vi "CaseStructure - Check If State Exist.vi"(8 "error in (no error)":errorcluster, 10 "Group Name":string, 11 "CaseStructure in":refnum<vi>) -> (0 "error out":errorcluster, 2 "Numeric":i32, 3 "CaseStructure out":refnum<vi>)   [LabVIEW 2017, in "csmHelper-CaseStructure.lvlib"]
doc: "-- <b>输入控件</b> --\n\n- <b>Group Name</b>:\n\n- <b>CaseStructure in</b>:\n\n-- <b>输出控件</b> --\n\n- <b>Numeric</b>:\n\n- <b>CaseStructure out</b>:"
uses:
  csmHelper-CaseStructure.lvlib
  Communicable State Machine.lvlib
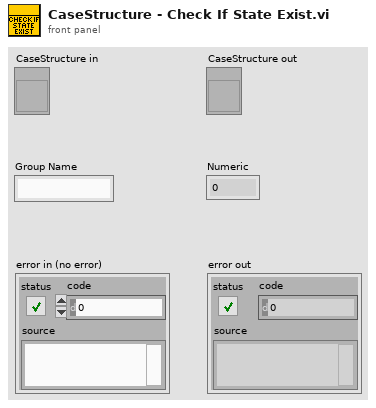
[diagram p1: front panel]
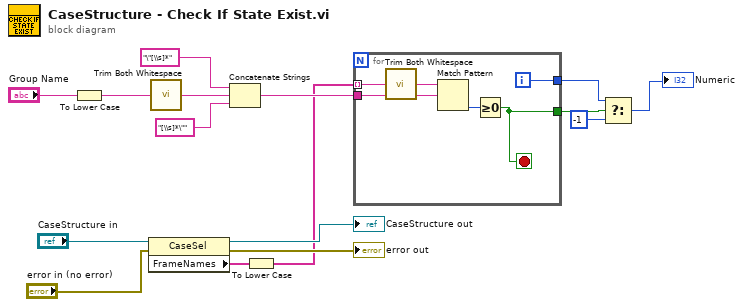
[diagram p0: block diagram]
diagram:
  n1 = To Lower Case(string="Group Name") -> (all lower case string=w7:string)
  n2 = property class="CaseSel"(reference="CaseStructure in", error in="error in (no error)") -> (reference out=→"CaseStructure out":refnum<vi>, error out=→"error out":errorcluster, "FrameNames"=w13:string[])
  n3 = call "Trim Both Whitespace.vi"("string"=w7) -> ("trimmed string"=w5:string)  [unwired: 1 in]
  n4 = Concatenate Strings("\"[\\s]*" ("regular expression"), w5, "[\\s]*\"" ("regular expression")) -> (w16:string)
  n5 = To Lower Case(string=w13) -> (all lower case string=w6:string[])
  n6 = for {
    tunnel: w6 -> [w22] mode=indexing
    tunnel: w16 -> [w20]
    tunnel: [w21] -> w3
    tunnel: [w17] -> w4
    i -> [w21]
    stop <- w17 stop-if-true
    n7 = call "Trim Both Whitespace.vi"("string"=w22) -> ("trimmed string"=w18:string)  [unwired: 1 in]
    n8 = Match Pattern(string=w18, regular expression=w20) -> (offset past match=w19:i32)  [unwired: 1 in, 3 out]
    n9 = Greater Or Equal To 0?(x=w19) -> (x >= 0?=w17:bool)
  }
  n10 = Select(t=w3, s=w4, f=-1) -> (s? t:f=→"Numeric":i32)
